vi "Initialize4WirexVDTParameters.vi"(6 "Specified Channel Ref List":T1[](array[typedef]) format="%.0x", 8 "error in":errorcluster, 9 "FPGA Session In":refnum<class "FPGA Interface Base.lvclass">, 11 "Device Reference in":T1 format="%.0x") -> (0 "error out":errorcluster, 1 "FPGA Session Out":refnum<class "FPGA Interface Base.lvclass">, 2 "4 Wire xVDT Parameters":T2[](array[typedef]), 3 "Device Reference out":T1 format="%.0x")   [LabVIEW 2011, in "Sensor Simulation Custom Device.lvlib"]
uses:
  Sensor Simulation Custom Device.lvlib
  <vilib>/NI Veristand/Custom Device API/Custom Device Item Ref.ctl
  TypeDefs/4 Wire xVDT Parameters.ctl
  <userlib>/_FPGA Interface Advanced Tools/FPGA Interface Base/FPGA Interface Base.lvclass
  TypeDefs/SensorType.ctl
  System Explorer/TypeDefs/xVDT.ctl
  <vilib>/rvi/DataTransferAndStorage/Container/Common/niFpgaDataTypeControl.ctl
  <userlib>/_FPGA Interface Advanced Tools/FPGA Interface Base/FPGA Interface Base.lvclass/FPGA Interface Base.ctl
  <vilib>/NI Veristand/Custom Device Tools/Custom Device Utility Library/NI VeriStand - Search for All Items by Property.vi
  Global.vi
  <vilib>/NI Veristand/Custom Device API/Get Item Property (Variant).vi
  <vilib>/NI Veristand/Custom Device API/Get Item Property (Double).vi
  <vilib>/Utility/error.llb/Error Cluster From Error Code.vi
  <vilib>/NI Veristand/Custom Device API/Custom Device API.lvlib
  <vilib>/NI Veristand/Custom Device Tools/Custom Device Utility Library/Custom Device Utility Library.lvlib
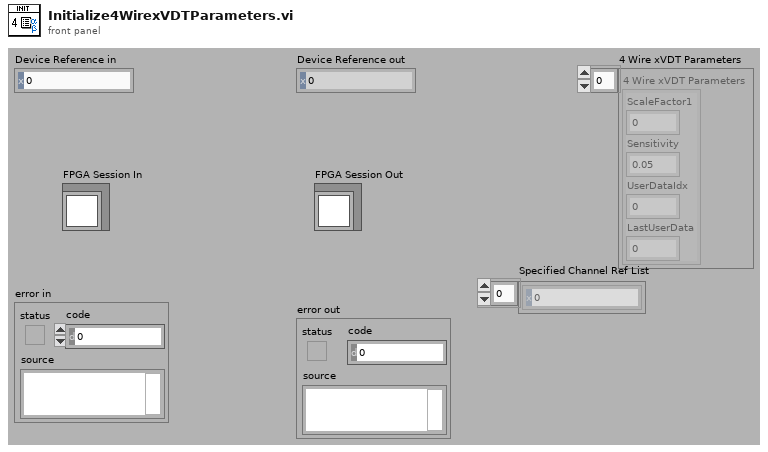
[diagram p1: front panel]
types:
  T1 = typedef "Custom Device API.lvlib/Custom Device Item Ref.ctl" = u64
  T2 = typedef "Sensor Simulation Custom Device.lvlib/4 Wire xVDT Parameters.ctl" = cluster{"ScaleFactor1":u32, "Sensitivity":dbl, "UserDataIdx":i32, "LastUserData":dbl}
  T3 = typedef "Sensor Simulation Custom Device.lvlib/SensorType.ctl" = enum16{"Resolver", "4 Wire xVDT", "5 Wire xVDT", "Invalid"}
  T4 = typedef "niFpgaDataTypeControl.ctl" = enum32{"Boolean", "I8", "I16", "I32", "I64", "U8", "U16", "U32", "U64", "FXP", "CustomControl"}
  T5 = typedef "Sensor Simulation Custom Device.lvlib/xVDT.ctl" = cluster{"ScaleFactor 1":string, "ScaleFactor 2":string, "#":string}
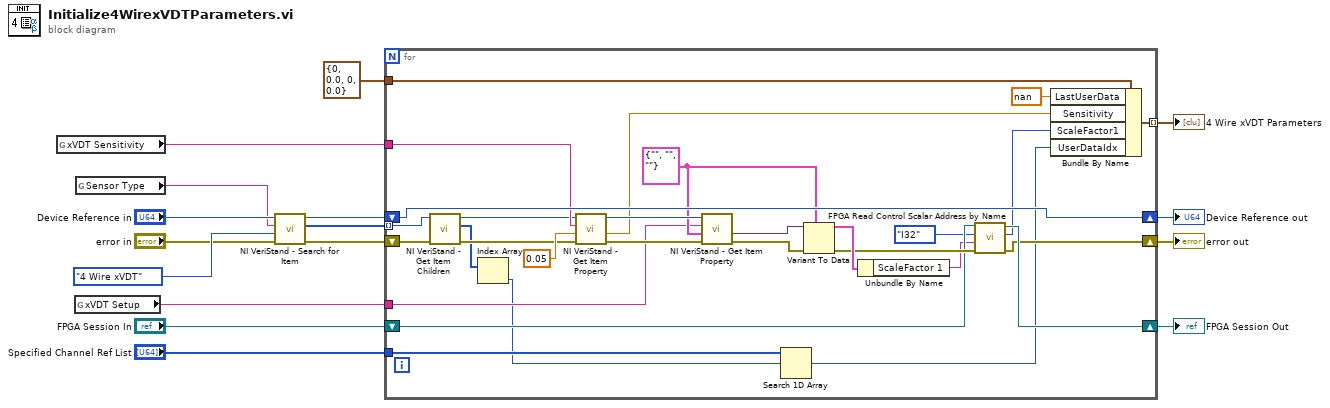
[diagram p0: block diagram]
diagram:
  n1 = global read "Global.vi" "xVDT Sensitivity"() -> (w4:string)
  n2 = global read "Global.vi" "xVDT Setup"() -> (w3:string)
  n3 = global read "Global.vi" "Sensor Type"() -> (w15:string)
  n4 = call-poly <vilib>:"NI VeriStand - Search for Item.vi"("error in"="error in", "Property Value"=SensorType."4 Wire xVDT" ("Sensor"), "Property Name"=w15, "Section Ref in"="Device Reference in") -> ("error out"=w6:errorcluster, "Item Refs"=w7:T1[], "Section Ref out"=w9:T1)  [unwired: 4 in, 1 out]
  n5 = for {
    shift-right: [w26] -> w11
    shift-left: w6 -> [w44]
    tunnel: w7 -> [w21] mode=indexing
    tunnel: T2 {"ScaleFactor1"=0, "Sensitivity"=0.0, "UserDataIdx"=0, "LastUserData"=0.0} ("4 Wire LVDT Parameters") -> [w37]
    tunnel: [w35] -> w12 mode=indexing
    shift-right: [w43] -> w13
    shift-left: w9 -> [w43]
    shift-right: [w29] -> w2
    shift-left: "FPGA Session In" -> [w30]
    tunnel: w4 -> [w33]
    tunnel: w3 -> [w32]
    tunnel: "Specified Channel Ref List" -> [w24]
    w39 = T5 {"ScaleFactor 1"="", "ScaleFactor 2"="", "#"=""} ("xVDT")
    n6 = call <vilib>:"NI VeriStand - Get Item Children.vi"("error in (no error)"=w44, "Item Ref in"=w21) -> ("error out"=w22:errorcluster, "Child Refs"=w19:T1[], "Item Ref out"=w20:T1)  [unwired: 6 in, 1 out]
    n7 = Index Array(array=w19) -> (element=w18:T1)  [unwired: 1 in]
    n8 = call-poly <vilib>:"NI VeriStand - Get Item Property.vi"("error in (no error)"=w22, "Default Value"=0.05, "Property Name"=w33, "Item Ref in"=w20) -> ("error out"=w34:errorcluster, "Value"=w36:dbl, "Item Ref out"=w42:T1)  [unwired: 4 in, 1 out]
    n9 = call-poly <vilib>:"NI VeriStand - Get Item Property.vi"("error in (no error)"=w34, "Default Value"=w39, "Property Name"=w32, "Item Ref in"=w42) -> ("error out"=w41:errorcluster, "Value"=w40:variant)  [unwired: 4 in, 2 out]
    n10 = Search 1D Array(1D array=w24, element=w18) -> (index of element=w23:i32)  [unwired: 1 in]
    n11 = Variant To Data(error in=w41, type=w39, Variant=w40) -> (data=w38:T5, error out=w31:errorcluster)
    n12 = Unbundle By Name(w38) -> ("ScaleFactor 1"=w28:string)
    n13 = call <userlib>:"FPGA Read Control Scalar Address by Name.vi"("error in (no error)"=w31, "Name"=w28, "Data Type"=niFpgaDataTypeControl."I32", "FPGA Interface Base in"=w30) -> ("error out"=w26:errorcluster, "Address"=w25:u32, "FPGA Interface Base out"=w29:refnum<class "FPGA Interface Base.lvclass">)  [unwired: 4 in, 1 out]
    n14 = Bundle By Name(cluster=w37, "LastUserData"=nan, "Sensitivity"=w36, "ScaleFactor1"=w25, "UserDataIdx"=w23) -> (w35:T2)
  }
  "error out" <- w11
  "Device Reference out" <- w13
  "4 Wire xVDT Parameters" <- w12
  "FPGA Session Out" <- w2
